vi "checkQueue.vi"(3 "Queue Max Size":i32=5, 4 "stop":bool, 5 "queue in":refnum<queue>) -> (2 "queue out":refnum<queue>)   [LabVIEW 2010]
doc: "Checks state of queue. Removes queue elements from front while queue size is greater than max. Initiates shutdown if stop is true."
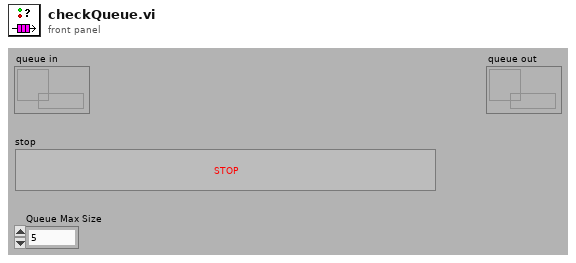
[diagram p1: front panel]
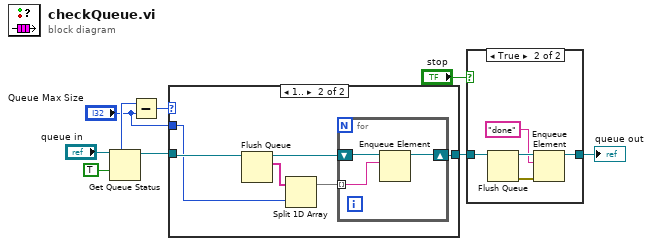
[diagram p0: block diagram]
diagram:
  n1 = Get Queue Status(queue="queue in", return elements? (F)=TRUE) -> (queue out=w4:refnum<queue>, # elements in queue=w6:i32)  [unwired: 1 in, 6 out]
  n2 = Subtract(x=w6, y="Queue Max Size") -> (x-y=w3:i32)
  n3 = case shown="1.." w3 {
    tunnel: [w10 w15] -> w8
    tunnel: w4 -> [w10 w14]
    tunnel: "Queue Max Size" -> [_ w12]
    frame Default {
    }
    frame 1.. {
      n4 = Flush Queue(queue=w14) -> (queue out=w16:refnum<queue>, remaining elements=w13:string[])  [unwired: 1 in, 1 out]
      n5 = Split 1D Array(array=w13, index=w12) -> (first subarray=w11:string[])  [unwired: 1 out]
      n6 = for {
        shift-right: [w18] -> w15
        shift-left: w16 -> [w19]
        tunnel: w11 -> [w17] mode=indexing
        n7 = Enqueue Element(queue=w19, element=w17) -> (queue out=w18:refnum<queue>)  [unwired: 2 in, 2 out]
      }
    }
  }
  n8 = case shown="True" "stop" {
    tunnel: w8 -> [w20 w22]
    tunnel: [w20 w21] -> w9
    frame False {
    }
    frame True {
      n9 = Flush Queue(queue=w22) -> (queue out=w25:refnum<queue>, error out=w24:errorcluster)  [unwired: 1 in, 1 out]
      n10 = Enqueue Element(queue=w25, element="done" ("regular expression"), error in (no error)=w24) -> (queue out=w21:refnum<queue>)  [unwired: 1 in, 2 out]
    }
  }
  "queue out" <- w9
